vi "di6ti.vi"() -> ()   [LabVIEW 2019]
panel:
  in  "pingjunshu":dbl[](array[numeric])
  in  "nianling":dbl[][](array[numeric])
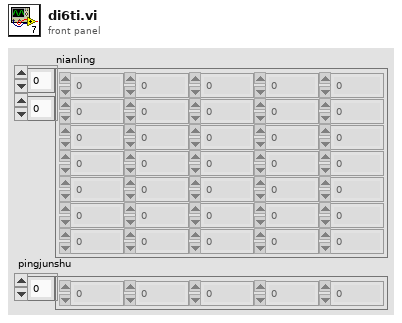
[diagram p1: front panel]
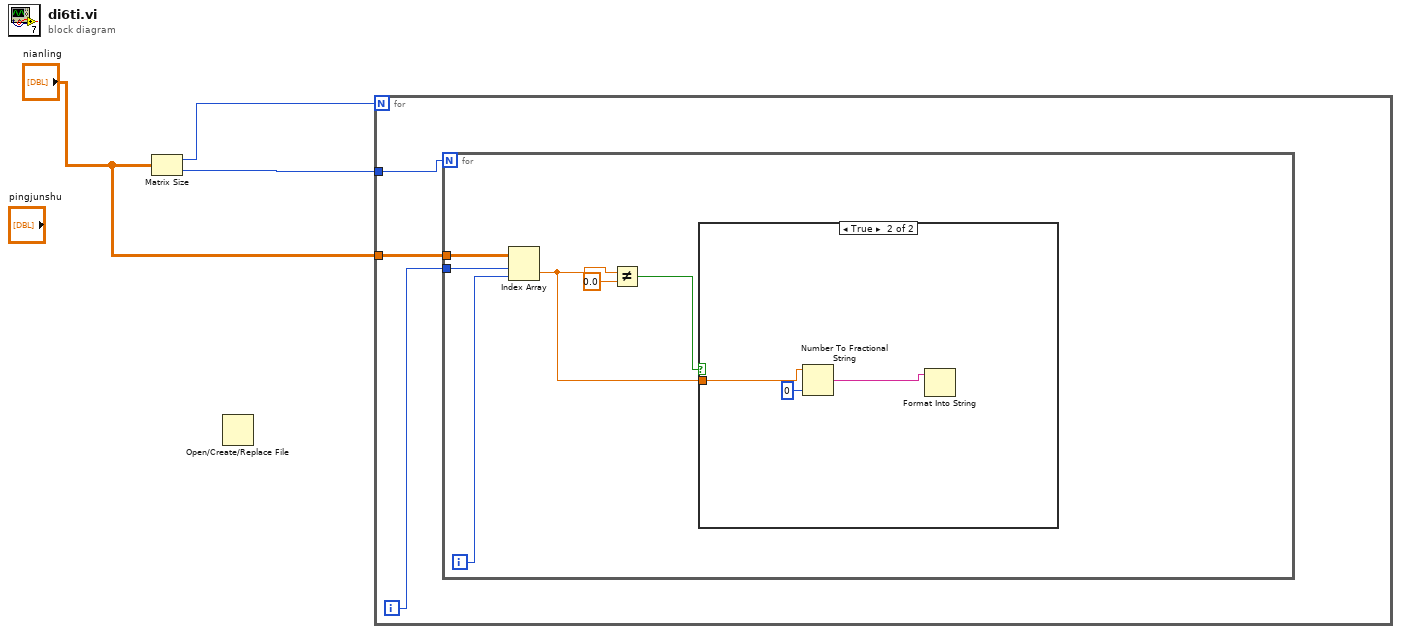
[diagram p0: block diagram]
diagram:
  n1 = Matrix Size(0:"nianling") -> (1:w3:i32, 2:w2:i32)
  n2 = Open/Create/Replace File() -> ()  [unwired: 6 in, 3 out]
  n3 = for {
    N: w3 -> [_]
    tunnel: w2 -> [w6]
    tunnel: "nianling" -> [w4]
    i -> [w5]
    n4 = for {
      N: w6 -> [_]
      tunnel: w5 -> [w12]
      tunnel: w4 -> [w10]
      i -> [w11]
      n5 = Index Array(array=w10, index (row)=w12, index (col)=w11) -> (element=w7:dbl)
      n6 = Not Equal?(x=w7, y=0.0) -> (x != y?=w8:bool)
      n7 = case shown="True" w8 {
        tunnel: w7 -> [_ w15]
        frame False {
        }
        frame True {
          n8 = Number To Fractional String(number=w15, precision (6)=i16 0) -> (F-format string=w13:string)  [unwired: 2 in]
          n9 = Format Into String(initial string=w13) -> ()  [unwired: 3 in, 2 out]
        }
      }
    }
  }
